vi "Write Max Number of Cores.vi"(8 "error in (no error)":errorcluster, 10 "Max Number of Cores":dbl, 11 "PC in":refnum<class "PC.lvclass">) -> (0 "error out":errorcluster, 3 "PC out":refnum<class "PC.lvclass">)   [LabVIEW 2017, in "PC.lvclass"]
uses:
  PC.lvclass
  PC.lvclass/PC.ctl
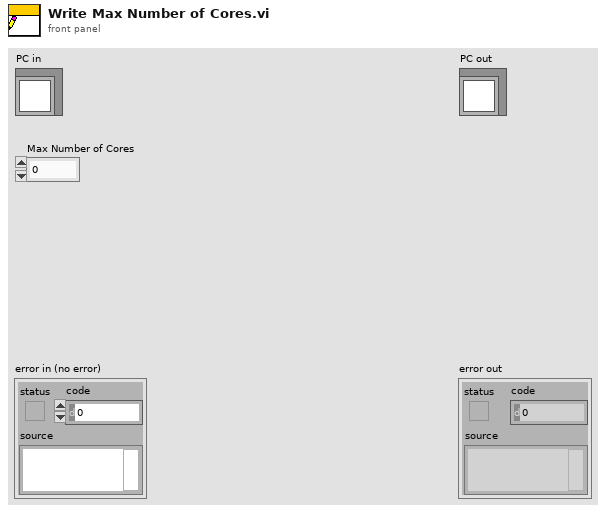
[diagram p1: front panel]
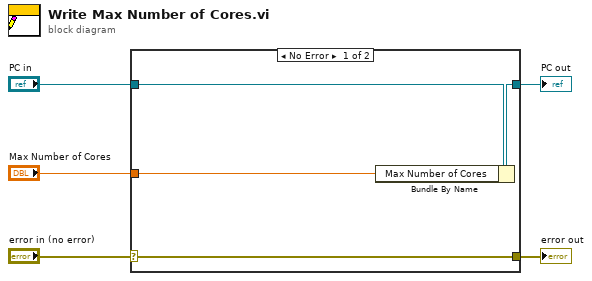
[diagram p0: block diagram]
diagram:
  n1 = case shown="No Error" "error in (no error)" {
    selector: "error in (no error)" -> [w9 w10]
    tunnel: [w9 w10] -> w4
    tunnel: [w7 w11] -> w2
    tunnel: "PC in" -> [w8 w11]
    tunnel: "Max Number of Cores" -> [w6 _]
    frame No Error {
      n2 = Bundle By Name(cluster=w8, "Max Number of Cores"=w6) -> (w7:refnum<class "PC.lvclass">)
    }
    frame Error {
    }
  }
  "error out" <- w4
  "PC out" <- w2
